vi "Calibration Cal IsNeeded RF Test Fetch Results.vi"(8 "error in (no error)":errorcluster, 11 "Template Tx Test in":refnum<class "niDTS Calibration Cal IsNeeded RF Test.lvclass">) -> (0 "error out":errorcluster, 2 "Default USL":T1, 3 "Template Tx Test out":refnum<class "niDTS Calibration Cal IsNeeded RF Test.lvclass">)   [LabVIEW 2015, in "niDTS Utilities.lvlib" / "niDTS Calibration Cal IsNeeded RF Test.lvclass"]
uses:
  niDTS Calibration Cal IsNeeded RF Test.lvclass
  Includes/niDTS Calibration Cal IsNeeded RF Test INC Results.ctl
  niDTS Calibration Cal IsNeeded RF Test.lvclass/niDTS Calibration Cal IsNeeded RF Test.ctl
  Calibration Cal IsNeeded Get InstDriver Handle in.vi
  Calibration Cal IsNeeded Get Ports.vi
  RiviInstDriver/niRfGeneralSettings/Objects/niRfGeneralSettings.lvclass
  niDTS Utilities.lvlib
  RiviInstDriver/InstDriver/Objects/InstDriver.lvclass
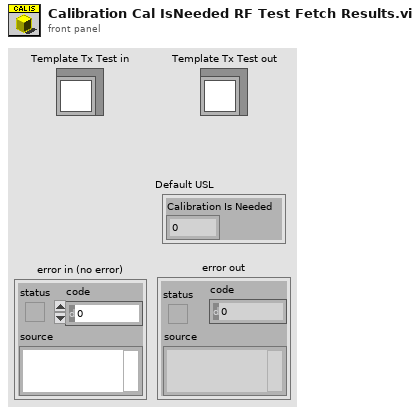
[diagram p1: front panel]
types:
  T1 = typedef "niDTS Utilities.lvlib/niDTS Calibration Cal IsNeeded RF Test INC Results.ctl" = cluster{"Calibration Is Needed":u8}
  T2 = typedef "niRfGeneralSettings.lvclass/niRfGeneralSettings INC Handle.ctl" = refnum<data-value>
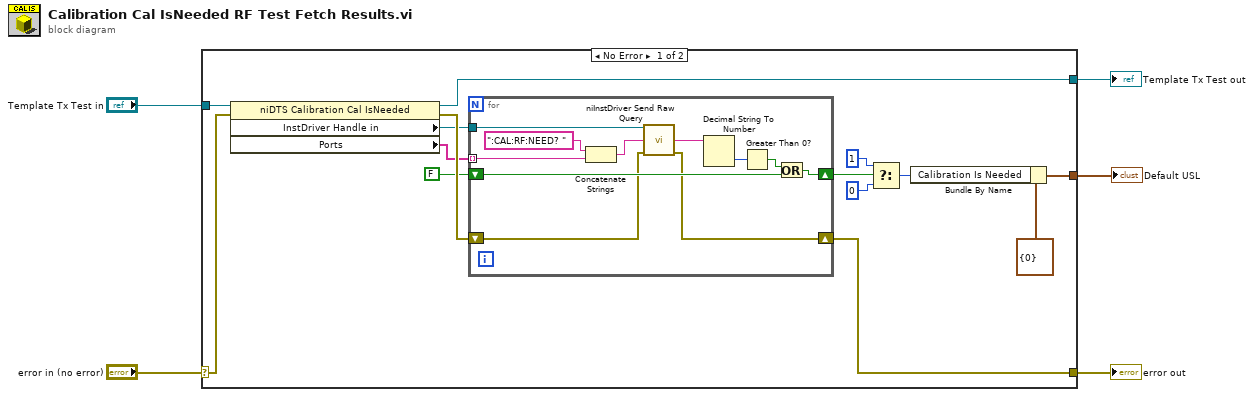
[diagram p0: block diagram]
diagram:
  n1 = case shown="No Error" "error in (no error)" {
    selector: "error in (no error)" -> [w13 w32]
    tunnel: [w15 w32] -> w4
    tunnel: [w14 w31] -> w2
    tunnel: "Template Tx Test in" -> [w18 w31]
    tunnel: [w17 _] -> w1
    frame No Error {
      n2 = property class="niDTS Calibration Cal IsNeeded "(reference=w18, error in=w13) -> (reference out=w14:refnum<class "niDTS Calibration Cal IsNeeded RF Test.lvclass">, error out=w16:errorcluster, "InstDriver Handle in"=w12:T2, "Ports"=w11:string[])
      n3 = for {
        tunnel: w11 -> [w25] mode=indexing
        shift-right: [w23] -> w15
        shift-left: w16 -> [w24]
        shift-right: [w29] -> w10
        shift-left: FALSE -> [w30]
        tunnel: w12 -> [w28]
        n4 = Concatenate Strings(":CAL:RF:NEED? ", w25) -> (w27:string)
        n5 = call "niInstDriver Send Raw Query.vi"("InstDriver Handle in"=w28, "Query"=w27, "error in (no error)"=w24) -> ("Response"=w22:string, "error out"=w23:errorcluster)  [unwired: 10 in, 1 out]
        n6 = Decimal String To Number(string=w22) -> (number=w21:i32)  [unwired: 2 in, 1 out]
        n7 = Greater Than 0?(x=w21) -> (x > 0?=w20:bool)
        n8 = Or(x=w20, y=w30) -> (x .or. y?=w29:bool)
      }
      n9 = Select(t=u8 1 ("Calibration Is Needed"), s=w10, f=u8 0 ("Calibration Is Needed")) -> (s? t:f=w7:u8)
      n10 = Bundle By Name(cluster=T1 {"Calibration Is Needed"=0} ("Default LSL"), "Calibration Is Needed"=w7) -> (w17:T1)
    }
    frame Error {
    }
  }
  "error out" <- w4
  "Template Tx Test out" <- w2
  "Default USL" <- w1
